vi "Read Temperature.vi"(8 "error in (no error)":errorcluster, 10 "SI":T1, 11 "TC01 in":refnum<class "TC01T.lvclass">) -> (0 "error out":errorcluster, 2 "Temperature":dbl, 3 "TC01 out":refnum<class "TC01T.lvclass">)   [LabVIEW 2018, in "TC01T.lvlib" / "TC01T.lvclass"]
uses:
  TC01T.lvclass
  builds/Thermocouple.lvlibp/Custom Controls/System Units.ctl
  builds/Thermocouple.lvlibp/Thermocouple.lvclass
  C:/Projects/LabVIEW/In-Progress/Jose Rivero-Diaz/builds/Thermocouple.lvlibp/Thermocouple.lvclass
  builds/Thermocouple.lvlibp
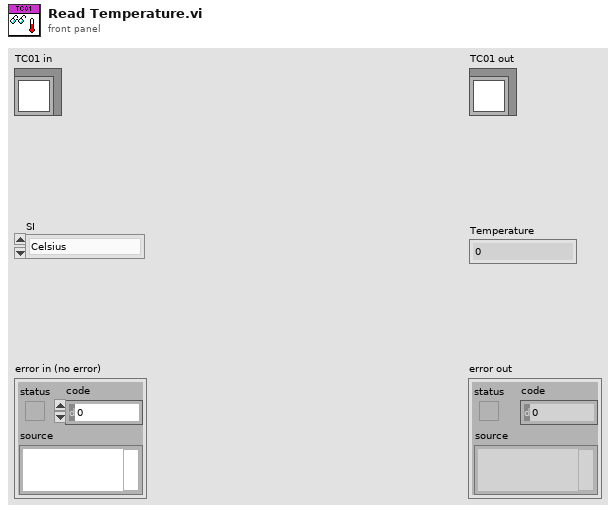
[diagram p1: front panel]
types:
  T1 = typedef "Thermocouple.lvlibp/System Units.ctl" = enum16{"Celsius", "Fahrenheit"}
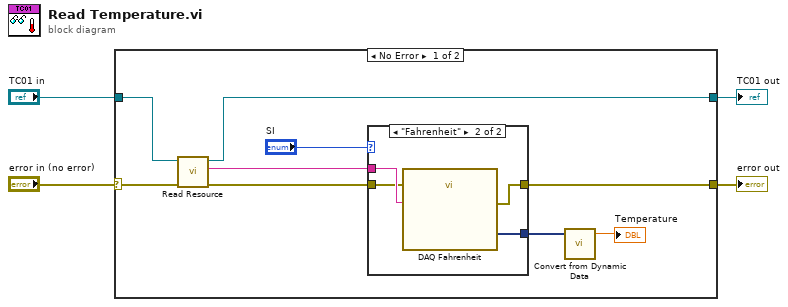
[diagram p0: block diagram]
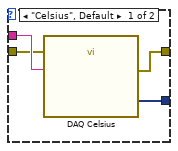
[diagram p2: hidden frame]
diagram:
  n1 = case shown="No Error" "error in (no error)" {
    selector: "error in (no error)" -> [w10 w22]
    tunnel: [w8 w22] -> w3
    tunnel: "TC01 in" -> [w12 w21]
    tunnel: [w11 w21] -> w1
    frame No Error {
      n2 = call "Read Resource.vi"("Thermocouple in"=w12) -> ("Resource"=w5:tag, "Thermocouple out"=w11:refnum<class "TC01T.lvclass">)  [unwired: 8 in, 1 out]
      n3 = case shown="\"Fahrenheit\"" "SI" {
        tunnel: w10 -> [w14 w18]
        tunnel: w5 -> [w15 w19]
        tunnel: [w16 w20] -> w7
        tunnel: [w13 w17] -> w8
        frame "Celsius", Default {
          n4 = call "DAQ Celsius"("error in"=w14, "device name"=w15) -> ("data"=w16:dynamicdata, "error out"=w13:errorcluster)  [unwired: 15 in, 1 out]
        }
        frame "Fahrenheit" {
          n5 = call "DAQ Fahrenheit"("error in"=w18, "device name"=w19) -> ("data"=w20:dynamicdata, "error out"=w17:errorcluster)  [unwired: 15 in, 1 out]
        }
      }
      n6 = call "Convert from Dynamic Data"("Dynamic Data Type"=w7) -> ("Scalar"=→"Temperature":dbl)  [unwired: 3 in]
    }
    frame Error {
    }
  }
  "error out" <- w3
  "TC01 out" <- w1
